vi "CountAtoms_LVFitting.vi"(0 "Cursor List":T4, 1 "Error In":errorcluster, 5 "Atom Image":dbl[][](graph), 7 "Experimental Variables":T3={"Pixel Size before binning (µm)"=6.0, "Imaging Wavelength (m)"=4.61e-07, "Isotope"=84, "1P1 Linewidth (MHz)"=30.5, "Imaging Detuning (MHz)"=0.0, "Software Bin Size"=1, "Exp. Trigger ON time (ms)"=0.0, "Path to spinapi.dll"=path "C:/SpinCore/SpinAPI/lib32/spinapi.dll", "PB clock_freq (MHz)"=100.0} {"Software Bin Size" items=["1"=1, "2"=2, "3"=3, "4"=4, "5"=5, "6"=6, "7"=7, "8"=8]; "Isotope" min=84 max=88; "Imaging Wavelength (m)" format="%#_6p"}, 9 "Background Image":dbl[][](graph), 11 "Drop Time":dbl=1e-06 min=1e-06 format="%#_6p", 12 "Trap Frequencies":T1) -> (2 "error out":errorcluster, 3 "Elapsed time ( ms)":u32, 4 "Number":dbl, 6 "OD":dbl[][](graph), 8 "Data Cuts":dbl[][](graph), 10 "Temperature (K) x":dbl format="%#_6p", 13 "Phase Space Density":dbl format="%#_3e", 14 "Best Fit Parameter Cluster":T2 {"Rot. Angle (deg)" format="%#.3g"; "Aspect Ratio" format="%#.3g"; "Y Width (um)" format="%#.3g"; "X Width (um)" format="%#.3g"; "Y Center (px)" format="%#.3g"; "X Center (px)" format="%#.3g"; "Amplitude (OD)" format="%#.3g"}, 15 "Temperature (K) y":dbl format="%#_6p")   [LabVIEW 2016]
uses:
  <vilib>/Utility/miscctls.llb/LVCursorListTypeDef.ctl
  Controls/ExperimentParameters/experimentalvariables.ctl
  Controls/2D Gaussian Fitting/Fit Parameter Cluster.ctl
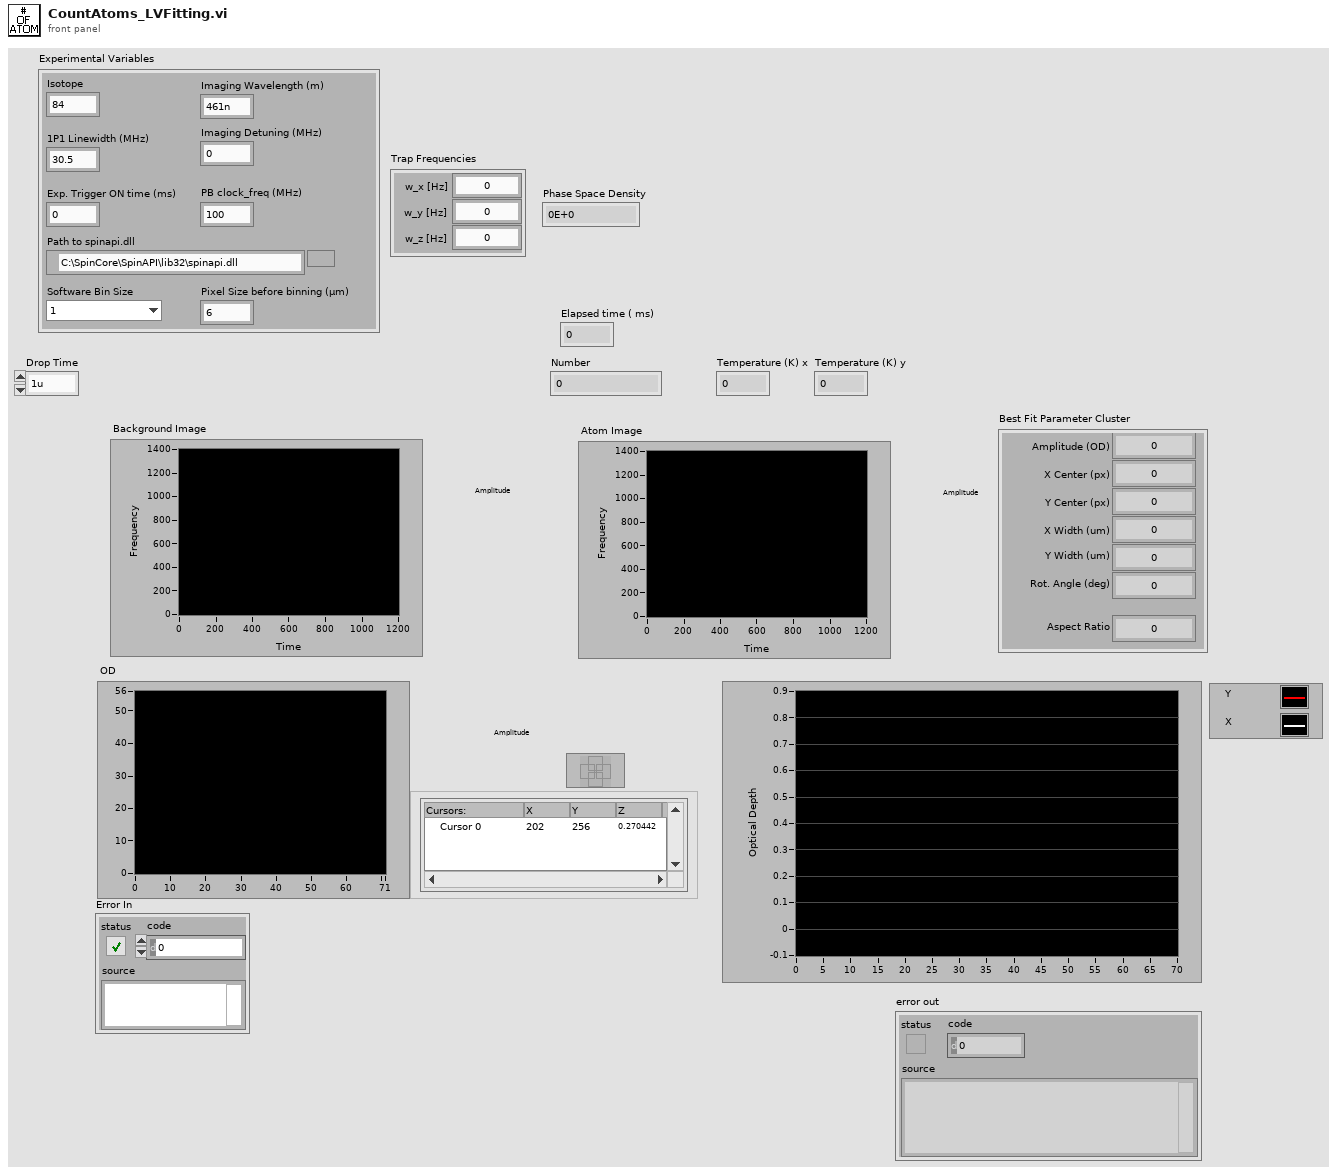
[diagram p1: front panel]
types:
  T1 = cluster{"w_x [Hz]":dbl, "w_y [Hz]":dbl, "w_z [Hz]":dbl}
  T2 = typedef "Fit Parameter Cluster.ctl" = cluster{"Amplitude (OD)":dbl, "X Center (px)":dbl, "Y Center (px)":dbl, " X Width (um)":dbl, "Y Width (um)":dbl, "Aspect Ratio":dbl, "Rot. Angle (deg)":dbl}
  T3 = typedef "experimentalvariables.ctl" = cluster{"Pixel Size before binning (µm)":dbl, "Imaging Wavelength (m)":dbl, "Isotope":i32, "1P1 Linewidth (MHz)":dbl, "Imaging Detuning (MHz)":dbl, "Software Bin Size":u16, "Exp. Trigger ON time (ms)":dbl, "Path to spinapi.dll":path, "PB clock_freq (MHz)":dbl}
  T4 = typedef "LVCursorListTypeDef.ctl" = cluster{"Name":string, "Color":u32, "Style":u8, "Point Style":u8, "Name Visible":bool, "Allow Drag":bool, "Cursor Mode":u32, "Plot":i32, "Index":i32, "Position":cluster{"X":dbl, "Y":dbl}, "X Scale":u32, "Y Scale":u32, "Watch Plots":i32[], "Watch All Plots":bool, "Plot Area":i32, "Label Offset":cluster{"X":dbl, "Y":dbl}}[]
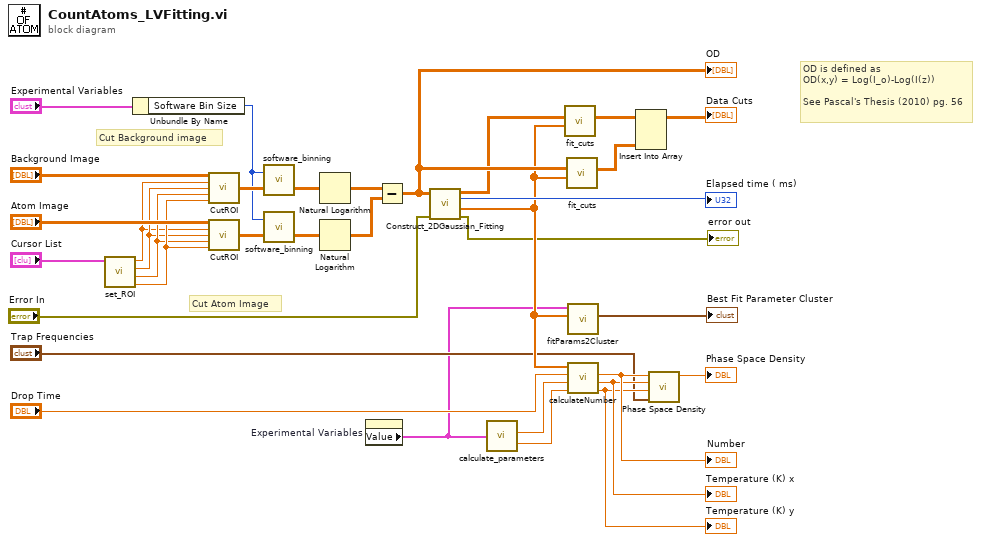
[diagram p0: block diagram]
diagram:
  # "OD is defined as \nOD(x,y) = Log(I_o)-Log(I(z))\n\nSee Pascal's Thesis (2010) pg. 56"
  # "Cut Atom Image"
  # "Cut Background image"
  n1 = call "set_ROI.vi"("Cursor List"="Cursor List") -> ("Row End"=w26:dbl, "RowStart"=w25:dbl, "ColEnd"=w24:dbl, "ColStart"=w23:dbl)  [unwired: 7 in]
  n2 = Unbundle By Name("Experimental Variables") -> ("Software Bin Size"=w17:u16)
  n3 = call "CutROI.vi"("Full Image In"="Background Image", "Col Start"=w23, "Col End"=w24, "Row Start"=w25, "Row End"=w26) -> ("Cut Image Out"=w21:dbl[][])  [unwired: 10 in]
  n4 = call "CutROI.vi"("Full Image In"="Atom Image", "Col Start"=w23, "Col End"=w24, "Row Start"=w25, "Row End"=w26) -> ("Cut Image Out"=w19:dbl[][])  [unwired: 10 in]
  n5 = call "software_binning.vi"("Input Array"=w21, "bin size"=w17) -> ("Binned Array"=w20:dbl[][])  [unwired: 1 in]
  n6 = call "software_binning.vi"("Input Array"=w19, "bin size"=w17) -> ("Binned Array"=w18:dbl[][])  [unwired: 1 in]
  n7 = Natural Logarithm(1:w20) -> (0:w28:dbl[][])
  n8 = Natural Logarithm(1:w18) -> (0:w27:dbl[][])
  n9 = property on="Experimental Variables" class="Clust (strict)"() -> ("Value"=w1:T3)  [unwired: 2 in, 2 out]
  n10 = Subtract(x=w28, y=w27) -> (x-y=w16:dbl[][])
  "OD" <- w16
  n11 = call "Construct_2DGaussian_Fitting.vi"("Error In"="Error In", "OD(2D)"=w16) -> ("error out"=→"error out":errorcluster, "best fit parameters"=w10:dbl[], "Elapsed time in ms"=→"Elapsed time ( ms)":u32, "Fit Image"=w14:dbl[][])  [unwired: 6 in]
  n12 = call "calculate_parameters.vi"("Experimental Variables"=w1) -> ("Effective Pixel Size (µm)"=w32:dbl, "Cross Section (m^2)"=w33:dbl)  [unwired: 8 in, 1 out]
  n13 = call "fit_cuts.vi"("Array"=w10, "Intensity Graph"=w14) -> ("Waveform Graph"=w13:dbl[][])  [unwired: 9 in]
  n14 = call "fit_cuts.vi"("Array"=w10, "Intensity Graph"=w16) -> ("Waveform Graph"=w12:dbl[][])  [unwired: 9 in]
  n15 = call "fitParams2Cluster.vi"("Experimental Variables"=w1, "Best fit parameters"=w10) -> ("Best Fit Parameter Cluster"=→"Best Fit Parameter Cluster":T2)  [unwired: 7 in]
  n16 = call "calculateNumber.vi"("Array"=w10, "Drop Time (s)"="Drop Time", "abs cross section (um^2)"=w33, "pixel size (um)"=w32) -> ("Number"=w6:dbl, "Temperature (K) x"=w5:dbl, "Temperature (K) y"=w4:dbl)  [unwired: 4 in]
  "Number" <- w6
  "Temperature (K) x" <- w5
  "Temperature (K) y" <- w4
  n17 = Insert Into Array(array=w13, new element=w12) -> (→"Data Cuts":dbl[][])  [unwired: 2 in]
  n18 = call "Phase Space Density.vi"("Trap Frequencies"="Trap Frequencies", "Temperature (K) y"=w4, "Temperature (K) x"=w5, "Number"=w6) -> ("Phase Space Density"=→"Phase Space Density":dbl)  [unwired: 7 in]
